vi "TLPM Find Resources.vi"(8 "error in (no error)":errorcluster {"code" format="%.0x"}, 11 "instrument handle":refnum<visa-resource-name>) -> (0 "error out":errorcluster {"code" format="%.0x"}, 2 "Resource Count":u32, 3 "instrument handle out":refnum<visa-resource-name>)   [LabVIEW 2017]
doc: "This VI finds all driver compatible devices attached to the PC and returns the number of found devices.\n\nNote:\n(1) The VI additionally stores information like system name about the found resources internally. This information can be retrieved with further VIs from the class, e.g. <Get Resource Description> and <Get Resource Information>."
uses:
  TLPM_64.dll
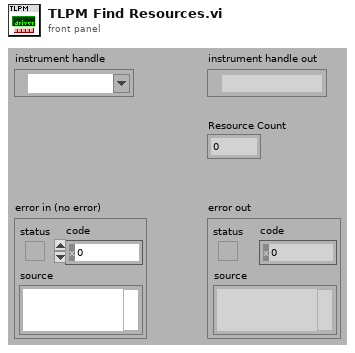
[diagram p1: front panel]
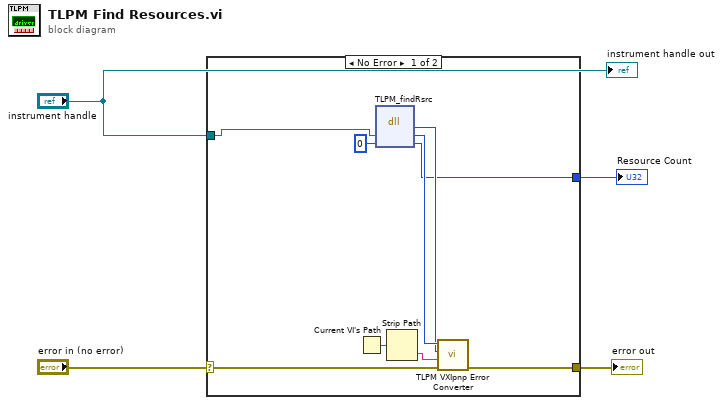
[diagram p0: block diagram]
diagram:
  n1 = case shown="No Error" "error in (no error)" {
    selector: "error in (no error)" -> [w8 w14]
    tunnel: [w7 w14] -> w4
    tunnel: "instrument handle" -> [w12 _]
    tunnel: [w5 _] -> w1
    frame No Error {
      n2 = Current VI's Path() -> (path=w13:path)
      n3 = dll-call lib="TLPM_64.dll" fn="TLPM_findRsrc"("Instrument Handle"=w12, "Resource Count"=u32 0) -> ("return type"=w10:i32, "Instrument Handle"=w11:u32, "Resource Count"=w5:u32)  [unwired: 3 in, 2 out]
      n4 = Strip Path(path=w13) -> (name=w9:string)  [unwired: 1 out]
      n5 = call "TLPM VXIpnp Error Converter.vi"("error in (no error)"=w8, "Name Of VI (\"\")"=w9, "CVI Error Code (0)"=w10, "instrument handle"=w11) -> ("error out"=w7:errorcluster)  [unwired: 6 in, 1 out]
    }
    frame Error {
    }
  }
  "error out" <- w4
  "Resource Count" <- w1
  "instrument handle out" <- "instrument handle"
